vi "HTTP Client.vi"() -> ()   [LabVIEW 2023]
uses:
  <vilib>/httpClient/LabVIEWHTTPClient.lvlib
panel:
  in  "stop":bool
  out "mid":dbl
  out "code":string
  in  "Combo Box":string(combo)
  out "effectiveDate":string
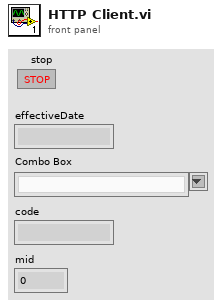
[diagram p1: front panel]
types:
  T1 = cluster{"table":string, "no":string, "effectiveDate":string, "rates":cluster{"currency":string, "code":string, "mid":dbl}[]}[]
  T2 = cluster{"table":string, "no":string, "effectiveDate":string, "rates":cluster{"currency":string, "code":string, "mid":dbl}[]}
  T3 = cluster{"currency":string, "code":string, "mid":dbl}[]
  T4 = cluster{"currency":string, "code":string, "mid":dbl}
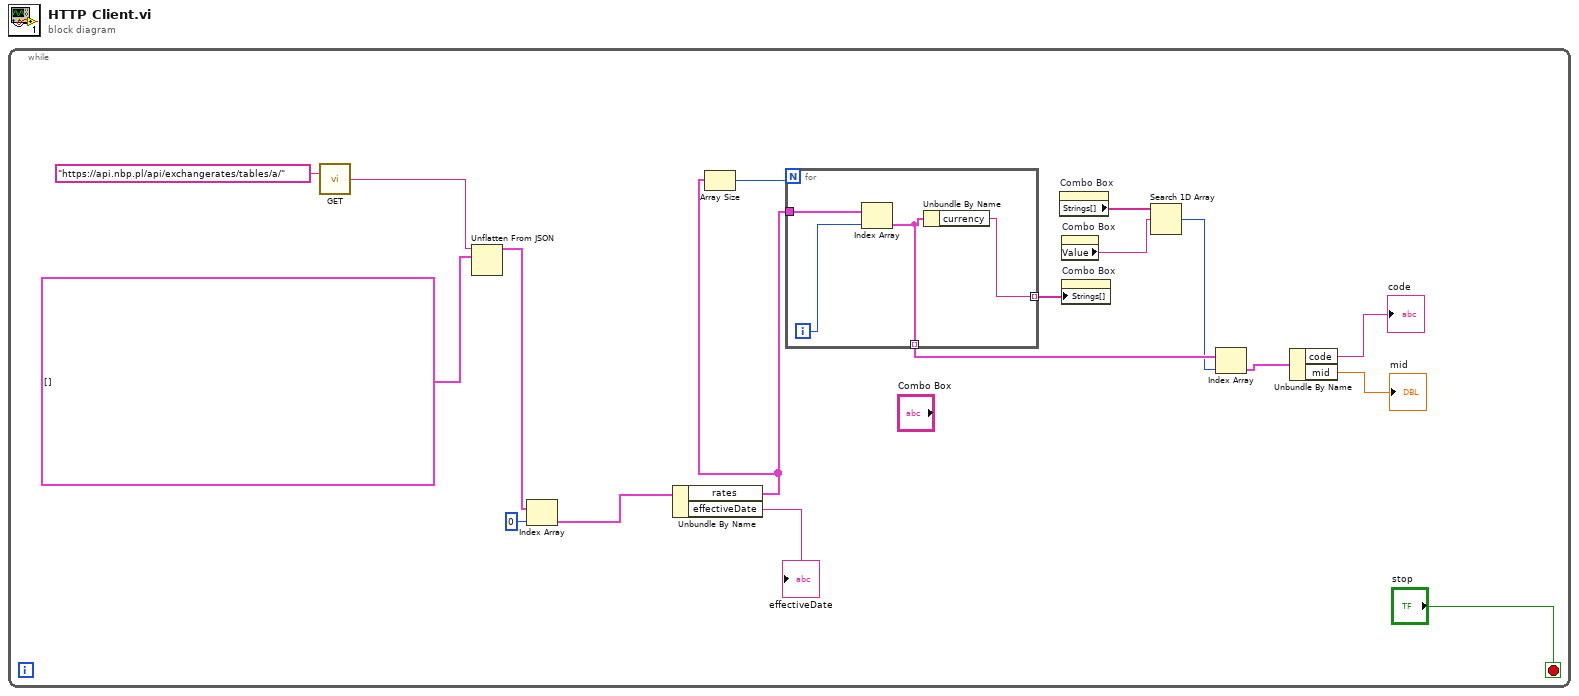
[diagram p0: block diagram]
diagram:
  n1 = while {
    stop <- "stop" stop-if-true
    n2 = call <vilib>:"GET.vi"("url"="https://api.nbp.pl/api/exchangerates/tables/a/") -> ("body"=w18:string)  [unwired: 11 in, 3 out]
    n3 = Unflatten From JSON(JSON string=w18, type and defaults=T1 []) -> (value=w1:T1)  [unwired: 5 in, 1 out]
    n4 = Index Array(array=w1, index=0) -> (element=w14:T2)
    n5 = Unbundle By Name(w14) -> ("rates"=w2:T3, "effectiveDate"=→"effectiveDate":string)
    n6 = Array Size(array=w2) -> (size(s)=w12:i32)
    n7 = for {
      N: w12 -> [_]
      tunnel: w2 -> [w21]
      tunnel: [w20] -> w9 mode=indexing
      tunnel: [w19] -> w8 mode=indexing
      i -> [w22]
      n8 = Index Array(array=w21, index=w22) -> (element=w19:T4)
      n9 = Unbundle By Name(w19) -> ("currency"=w20:string)
    }
    n10 = property on="Combo Box" class="CmbBox"() -> ("Strings[]"=w10:string[])  [unwired: 2 in, 2 out]
    n11 = property on="Combo Box" class="CmbBox"() -> ("Value"=w11:string)  [unwired: 2 in, 2 out]
    n12 = property on="Combo Box" class="CmbBox"("Strings[]"=w9) -> ()  [unwired: 2 in, 2 out]
    n13 = Search 1D Array(1D array=w10, element=w11) -> (index of element=w7:i32)  [unwired: 1 in]
    n14 = Index Array(array=w8, index=w7) -> (element=w6:T4)
    n15 = Unbundle By Name(w6) -> ("code"=→"code":string, "mid"=→"mid":dbl)
  }
